vi "Equals.vi"(1 "comparable 2":refnum<class "String With Equals.lvclass">, 2 "comparable 1":refnum<class "String With Equals.lvclass">) -> (0 "less?":bool)   [LabVIEW 2023, in "String With Equals.lvclass"]
doc: "Returns whether <b>Comparable 1</b> is less than, equal to, or greater than <b>Comparable 2</b>."
uses:
  String With Equals.lvclass
  String With Equals.lvclass/String With Equals.ctl
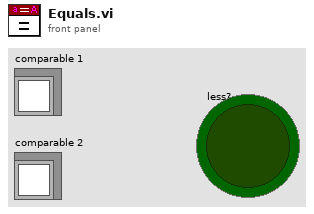
[diagram p1: front panel]
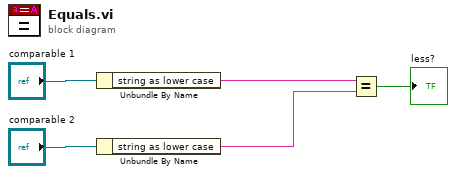
[diagram p0: block diagram]
diagram:
  n1 = Unbundle By Name("comparable 1") -> ("string as lower case"=w2:string)
  n2 = Unbundle By Name("comparable 2") -> ("string as lower case"=w1:string)
  n3 = Equal?(x=w2, y=w1) -> (x = y?=→"less?":bool)
